vi "CheckClientNumber.vi"(9 "Receive 2":T1, 10 "ID Module":i32, 11 "data in":string) -> (3 "Receive":T1)   [LabVIEW 2020, in "TCP_Client.lvlib"]
uses:
  TCP_Client.lvlib
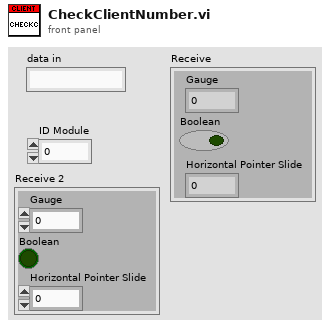
[diagram p1: front panel]
types:
  T1 = cluster{"Gauge":dbl, "Boolean":bool, "Horizontal Pointer Slide":dbl}
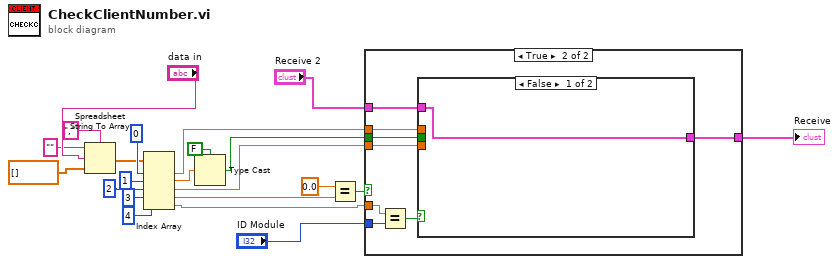
[diagram p0: block diagram]
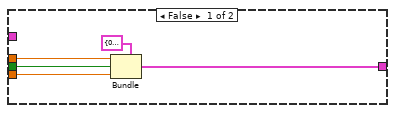
[diagram p2: hidden frame]
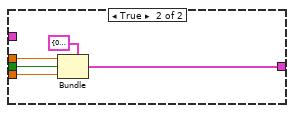
[diagram p3: hidden frame]
diagram:
  n1 = Spreadsheet String To Array(delimiter (Tab)=",", format string="", spreadsheet string="data in", array type (2D Dbl)=dbl[] []) -> (array=w8:dbl[])
  n2 = Index Array(array=w8, index #1=0 ("index"), index #2=1 ("index"), index #3=2 ("index"), index #4=3 ("index"), index #5=4 ("index")) -> (element #1=w9:dbl, element #2=w11:dbl, element #3=w10:dbl, element #4=w6:dbl, element #5=w3:dbl)
  n3 = Type Cast(type=FALSE, x=w11) -> (*(type *) &x=w12:bool)
  n4 = Equal?(x=0.0, y=w6) -> (x = y?=w7:bool)
  n5 = case shown="True" w7 {
    tunnel: w12 -> [w26 w35]
    tunnel: w10 -> [w25 w34]
    tunnel: w9 -> [w24 w33]
    tunnel: [w23 w32] -> w4
    tunnel: w3 -> [_ w29]
    tunnel: "ID Module" -> [_ w30]
    tunnel: "Receive 2" -> [_ w28]
    frame False {
      n6 = Bundle(cluster=T1 {"Gauge"=0.0, "Boolean"=FALSE, "Horizontal Pointer Slide"=5.0} ("Receive"), "Gauge"=w24, "Boolean"=w26, "Horizontal Pointer Slide"=w25) -> (w23:T1)
    }
    frame True {
      n7 = Equal?(x=w29, y=w30) -> (x = y?=w31:bool)
      n8 = case shown="False" w31 {
        tunnel: w35 -> [_ w40]
        tunnel: w34 -> [_ w39]
        tunnel: w33 -> [_ w38]
        tunnel: [w36 w37] -> w32
        tunnel: w28 -> [w36 _]
        frame False {
        }
        frame True {
          n9 = Bundle(cluster=T1 {"Gauge"=0.0, "Boolean"=FALSE, "Horizontal Pointer Slide"=5.0} ("Receive"), "Gauge"=w38, "Boolean"=w40, "Horizontal Pointer Slide"=w39) -> (w37:T1)
        }
      }
    }
  }
  "Receive" <- w4
